vi "Camera_TakePicture.vi"(8 "error in (no error)":errorcluster, 9 "appended path":path, 10 "Handle":refnum<k24>, 11 ".NET Refnum in":refnum<k24>) -> (0 "error out":errorcluster, 3 ".NET Refnum out":refnum<k24>)   [LabVIEW 2020]
uses:
  C:/Program Files/Thorlabs/Scientific Imaging/DCx Camera Support/Develop/DotNet/uc480DotNet.dll
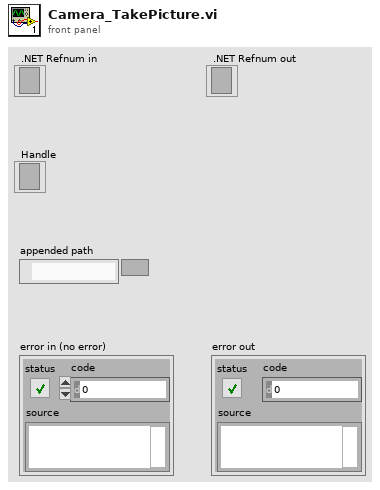
[diagram p1: front panel]
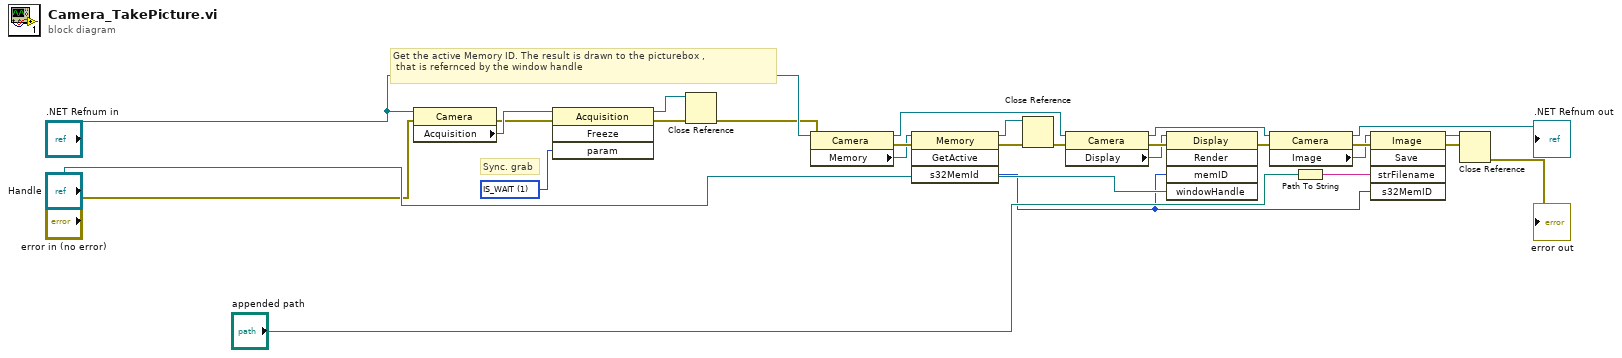
[diagram p0: block diagram]
diagram:
  w13 = 1 items=["IS_DONT_WAIT", "IS_WAIT"] ("Wait")
  # "Sync. grab"
  # "Get the active Memory ID. The result is drawn to the picturebox ,\n that is refernced by the window handle"
  n1 = property class="Camera"(reference=".NET Refnum in", error in="error in (no error)") -> (error out=w11:errorcluster, "Acquisition"=w12:refnum<k24>)  [unwired: 1 out]
  n2 = invoke class="Acquisition" method="Freeze"(reference=w12, error in=w11, "param"=w13) -> (reference out=w9:refnum<k24>, error out=w10:errorcluster)  [unwired: 1 in, 2 out]
  n3 = Close Reference(reference=w9, error in (no error)=w10) -> (error out=w14:errorcluster)
  n4 = property class="Camera"(reference=".NET Refnum in", error in=w14) -> (reference out=w8:refnum<k24>, error out=w2:errorcluster, "Memory"=w1:refnum<k24>)
  n5 = invoke class="Memory" method="GetActive"(reference=w1, error in=w2) -> (reference out=w4:refnum<k24>, error out=w5:errorcluster, "s32MemId"=w17:i32)  [unwired: 2 in, 1 out]
  n6 = Close Reference(reference=w4, error in (no error)=w5) -> (error out=w6:errorcluster)
  n7 = property class="Camera"(reference=w8, error in=w6) -> (reference out=w15:refnum<k24>, error out=w7:errorcluster, "Display"=w3:refnum<k24>)
  n8 = invoke class="Display" method="Render"(reference=w3, error in=w7, "memID"=w17, "windowHandle"="Handle") -> (error out=w18:errorcluster)  [unwired: 1 in, 4 out]
  n9 = property class="Camera"(reference=w15, error in=w18) -> (reference out=→".NET Refnum out":refnum<k24>, error out=w19:errorcluster, "Image"=w16:refnum<k24>)
  n10 = Path To String(path="appended path") -> (string=w21:string)
  n11 = invoke class="Image" method="Save"(reference=w16, error in=w19, "strFilename"=w21, "s32MemID"=w17) -> (reference out=w26:refnum<k24>, error out=w27:errorcluster)  [unwired: 1 in, 3 out]
  n12 = Close Reference(reference=w26, error in (no error)=w27) -> (error out=→"error out":errorcluster)
